vi "Untitled 1.vi"() -> ()   [LabVIEW 2016]
uses:
  builds/UnicornMain/UnicornRIO1/ROS for LabVIEW/home/lvuser/natinst/bin/user.lib/ROS for LabVIEW Software/ROS/Code/Console/Servers/ServerSubs/TopicDef.ctl
  builds/UnicornMain/UnicornRIO1/ROS for LabVIEW/home/lvuser/natinst/bin/user.lib/ROS for LabVIEW Software/ROS/Code/SubVIs/_ROSDirection.ctl
  builds/UnicornMain/UnicornRIO1/ROS for LabVIEW/home/lvuser/natinst/bin/user.lib/ROS for LabVIEW Software/ROS/MessageBuilding/std_msgs/subs/i32Scalar.vi
panel:
  in  "stop":bool
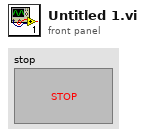
[diagram p1: front panel]
types:
  T1 = typedef "TopicDef.ctl" = cluster{"Topic":string, "Type":string, "Action":T2, "Update (ms)":u16, "queue size":u16}
  T2 = typedef "_ROSDirection.ctl" = enum16{"Node", "Publisher", "Subscriber", "ServiceClient", "ServiceProvider"}
  T3 = typedef "_ROSControl.ctl" = cluster{"topic port":u16, "Node":string, "topic":string, "type":string, "node port":u16, "error ":errorcluster, "Direction":T2, "Update (ms)":u16, "FIFO size":u16}
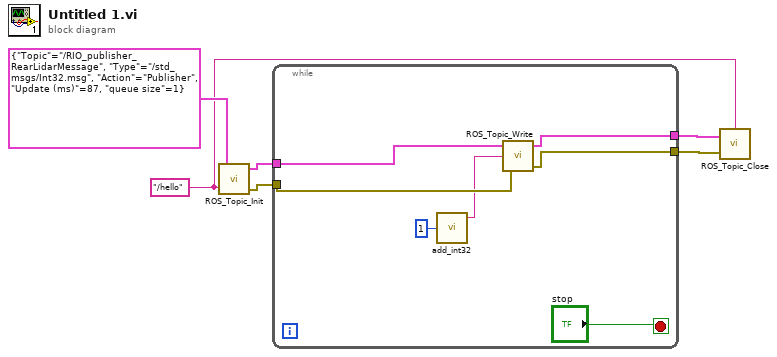
[diagram p0: block diagram]
diagram:
  w1 = "/hello" ("node")
  n1 = call "ROS_Topic_Init.vi"("Definitions"=T1 {"Topic"="/RIO_publisher_RearLidarMessage", "Type"="/std_msgs/Int32.msg", "Action"=enum."Publisher", "Update (ms)"=87, "queue size"=1}, "node"=w1) -> ("ROS out"=w5:T3, "error out"=w4:errorcluster)  [unwired: 1 in]
  n2 = while {
    tunnel: w5 -> [w13]
    tunnel: w4 -> [w12]
    tunnel: [w9] -> w3
    tunnel: [w8] -> w2
    stop <- "stop" stop-if-true
    n3 = call-poly "add_int32.vi"("Numeric"=1) -> ("msg out"=w10:string)  [unwired: 4 in]
    n4 = call "ROS_Topic_Write.vi"("error in (no error)"=w12, "Msg in"=w10, "ROS in"=w13) -> ("error out"=w8:errorcluster, "ROS out"=w9:T3)  [unwired: 1 in]
  }
  n5 = call "ROS_Topic_Close.vi"("error in"=w2, "ROS in"=w3, "node"=w1) -> ()  [unwired: 1 in, 1 out]
